vi "Property Tree_Populate Trees.vi"(4 "Close Items":bool, 5 "VI Ref":refnum<vi>, 6 "Filter":string, 7 "Action":T3, 8 "Error In":errorcluster, 9 "Tree Refs":refnum<vi>[](array[refnum]), 10 "Show":T1, 11 "Properties for Tree In":T2(array[cluster])) -> (0 "error out":errorcluster)   [LabVIEW 2023]
uses:
  controls/action enum.ctl
  Libraries/Tree Handler/Tree Handlr.lvlib
panel:
  out "exe time (ms)":u32
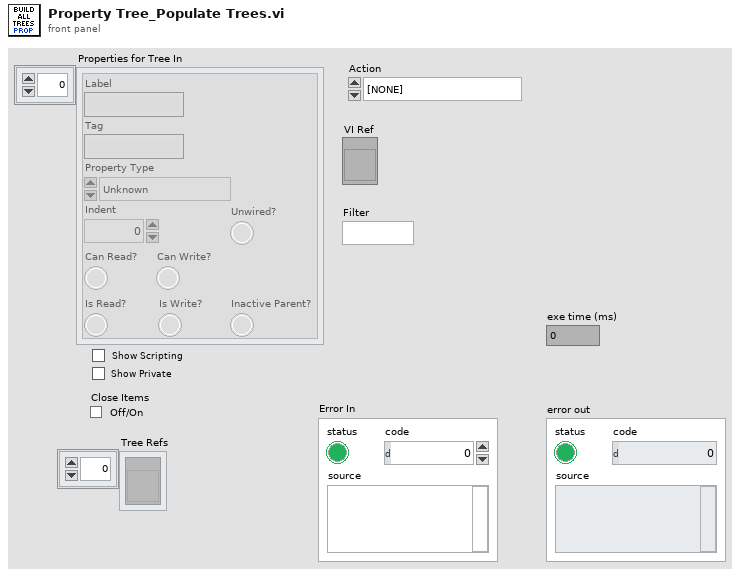
[diagram p1: front panel]
types:
  T1 = cluster{"Show Scripting":bool, "Show Private":bool}
  T2 = cluster{"Label":string, "Tag":string, "Property Type":enum16{"Unknown", "Base", "Scripting", "Private", "Deprecated", "None", "Divider"}, "Indent":u16, "Can Read?":bool, "Can Write?":bool, "Is Read?":bool, "Is Write?":bool, "Inactive Parent?":bool, "Unwired?":bool}[]
  T3 = typedef "action enum.ctl" = enum16{"[NONE]", "APP_SEPARATOR", "Wire Bundle", "Wire Unbundle", "Terminal Unbundle", "Terminal Bundle", "Bundler Move Up", "Bundler Move Down", "Bundler Insert", "Bundler Remove", "Bundler Remove Unwired", "Bundler Reorder", "In Place Insert", "In Place Remove", "In Place Remove Unwired", "In Place Reorder", "Wire Properties", "Wire Method", "Terminal Properties", "Terminal Method", "Property Move Up", "Property Move Down", "Properties Insert", "Properties Remove", "Properties Remove Unwired", "Properties Reorder", "Method Change", "Class For Constant", "Class For Control", "Class For Node", "Class Name to Clipboard"}
  T4 = cluster{"Show":cluster{"Show Scripting":bool, "Show Private":bool}, "Filter":string}
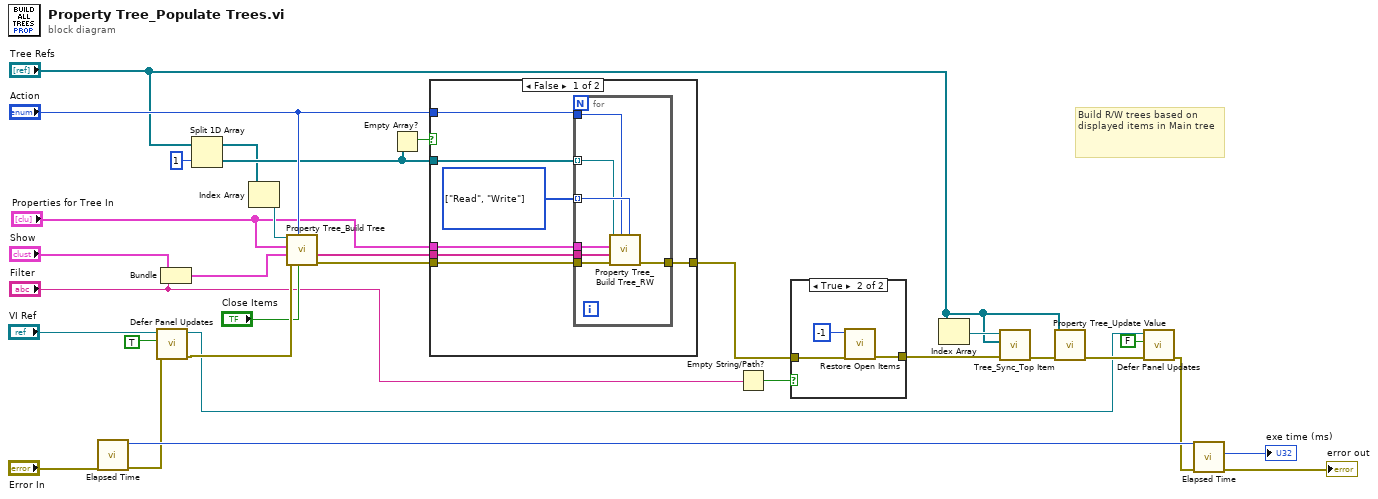
[diagram p0: block diagram]
diagram:
  # "Build R/W trees based on displayed items in Main tree"
  n1 = call "Elapsed Time.vi"("error in"="Error In") -> ("error out"=w9:errorcluster, "millisecond timer value"=w25:u32)  [unwired: 6 in, 3 out]
  n2 = call "Defer Panel Updates.vi"("error in (no error)"=w9, "Defer Panel Updates [T]"=TRUE, "VI Ref"="VI Ref") -> ("error out"=w30:errorcluster, "VI Ref Out"=w26:refnum<vi>)  [unwired: 7 in]
  n3 = Bundle("Show"="Show", "Filter"="Filter") -> (w22:T4)  [unwired: 1 in]
  n4 = Split 1D Array(array="Tree Refs", index=1) -> (first subarray=w7:refnum<vi>[], second subarray=w15:refnum<vi>[])
  n5 = Index Array(array=w7) -> (element=w16:refnum<vi>)  [unwired: 1 in]
  n6 = call "Property Tree_Build Tree.vi"("Close Items"="Close Items", "Action"="Action", "error in"=w30, "Filter"=w22, "Properties for Tree"="Properties for Tree In", "Tree Ref"=w16) -> ("error out"=w19:errorcluster, "Displayed Items"=w20:string[])  [unwired: 2 in, 2 out]
  n7 = Empty Array?(array=w15) -> (empty?=w14:bool)
  n8 = case shown="False" w14 {
    tunnel: w20 -> [w38 _]
    tunnel: w19 -> [w37 w46]
    tunnel: [w36 w46] -> w6
    tunnel: "Properties for Tree In" -> [w35 _]
    tunnel: "Action" -> [w33 _]
    tunnel: w15 -> [w32 _]
    frame False {
      w34 = enum16{"Main", "Write", "Read"}[] [enum."Read", enum."Write"] items=["Main", "Write", "Read"] ("Tree Type")
      n9 = for {
        tunnel: w38 -> [w45]
        tunnel: w35 -> [w42]
        tunnel: w37 -> [w44]
        tunnel: [w43] -> w36
        tunnel: w34 -> [w41] mode=indexing
        tunnel: w33 -> [w40]
        tunnel: w32 -> [w39] mode=indexing
        n10 = call "Property Tree_Build Tree_RW.vi"("Tree Type"=w41, "Action"=w40, "error in"=w44, "Displayed Items"=w45, "Properties for Tree"=w42, "Tree Ref"=w39) -> ("error out"=w43:errorcluster)  [unwired: 3 in, 2 out]
      }
    }
    frame True {
    }
  }
  n11 = Empty String/Path?(string/path="Filter") -> (empty?=w3:bool)
  n12 = case shown="True" w3 {
    tunnel: w6 -> [w47 w49]
    tunnel: [w47 w48] -> w5
    frame False {
    }
    frame True {
      n13 = call "Restore Open Items.vi"("error in"=w49, "Module ID"=-1) -> ("error out"=w48:errorcluster)  [unwired: 9 in]
    }
  }
  n14 = Index Array(array="Tree Refs") -> (element=w2:refnum<vi>)  [unwired: 1 in]
  n15 = call "Tree_Sync_Top Item.vi"("error in"=w5, "All Tree Control Refs"="Tree Refs", "Changed Tree Control Ref"=w2) -> ("error out"=w8:errorcluster)  [unwired: 8 in]
  n16 = call "Property Tree_Update Value.vi"("error in"=w8, "Tree Ref Array Out"="Tree Refs") -> ("error out"=w28:errorcluster)  [unwired: 9 in]
  n17 = call "Defer Panel Updates.vi"("error in (no error)"=w28, "Defer Panel Updates [T]"=FALSE, "VI Ref"=w26) -> ("error out"=w12:errorcluster)  [unwired: 7 in, 1 out]
  n18 = call "Elapsed Time.vi"("error in"=w12, "past time"=w25) -> ("error out"=→"error out":errorcluster, "elapsed time (ms)"=→"exe time (ms)":u32)  [unwired: 5 in, 3 out]
